vi "Read Header.vi"(8 "error in (no error)":errorcluster, 11 "Update Header MSG in":refnum<class "Update Header MSG.lvclass">) -> (0 "error out":errorcluster, 2 "Header":string, 3 "Update Header MSG out":refnum<class "Update Header MSG.lvclass">)   [LabVIEW 2017, in "File Library.lvlib" / "Update Header MSG.lvclass"]
uses:
  Update Header MSG.lvclass
  Update Header MSG.lvclass/Update Header MSG.ctl
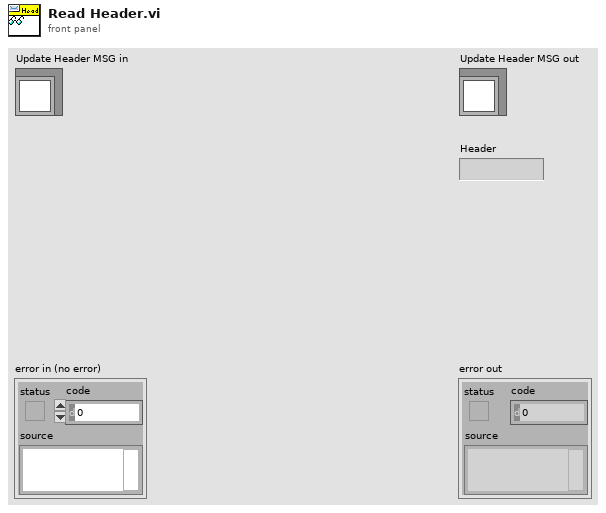
[diagram p1: front panel]
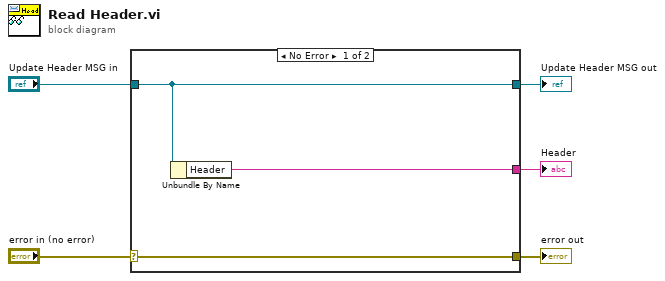
[diagram p0: block diagram]
diagram:
  n1 = case shown="No Error" "error in (no error)" {
    selector: "error in (no error)" -> [w8 w9]
    tunnel: [w8 w9] -> w4
    tunnel: [w7 w10] -> w2
    tunnel: "Update Header MSG in" -> [w7 w10]
    tunnel: [w6 _] -> w1
    frame No Error {
      n2 = Unbundle By Name(w7) -> ("Header"=w6:string)
    }
    frame Error {
    }
  }
  "error out" <- w4
  "Update Header MSG out" <- w2
  "Header" <- w1
